vi "Convert CAN Log Files.vi"() -> ()   [LabVIEW 2010, in "CAN Log Transfer and Convert.lvlib"]
uses:
  CAN Log Transfer and Convert.lvlib
  NICAN Warning.ctl
  Stop FGV Commands.ctl
  Global.vi
panel:
  out "CAN Warning":T1=TRUE
  in  "Text format":enum32{"NI-CAN", "NI-XNET"}(radio)
  in  "Destination directory":path
  in  "Recursive?":bool=TRUE
  in  "Directory of NCL files":path
  out "Progress":u8(slide) scale=0.0..100.0
  in  "Abort":bool
  in  "Start":bool
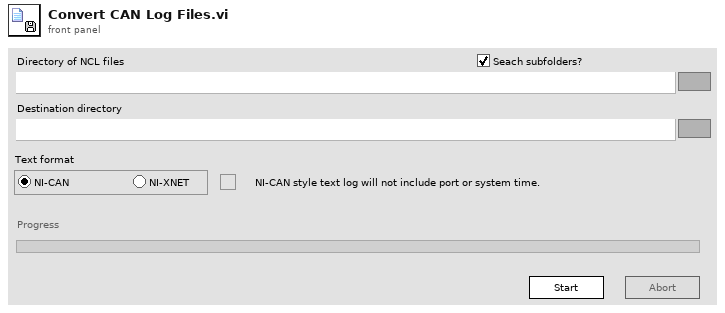
[diagram p1: front panel]
types:
  T1 = typedef "CAN Log Transfer and Convert.lvlib/NICAN Warning.ctl" = bool
  T2 = typedef "CAN Log Transfer and Convert.lvlib/Stop FGV Commands.ctl" = enum16{"Write", "Read", "Reset"}
  T3 = enum8{"Enabled", "Disabled", "Disabled and Grayed Out"}
  T4 = enum32{"invalid app kind", "Development System", "Run Time System", "Student Edition", "Embedded LabVIEW", "Evaluation", "Custom"}
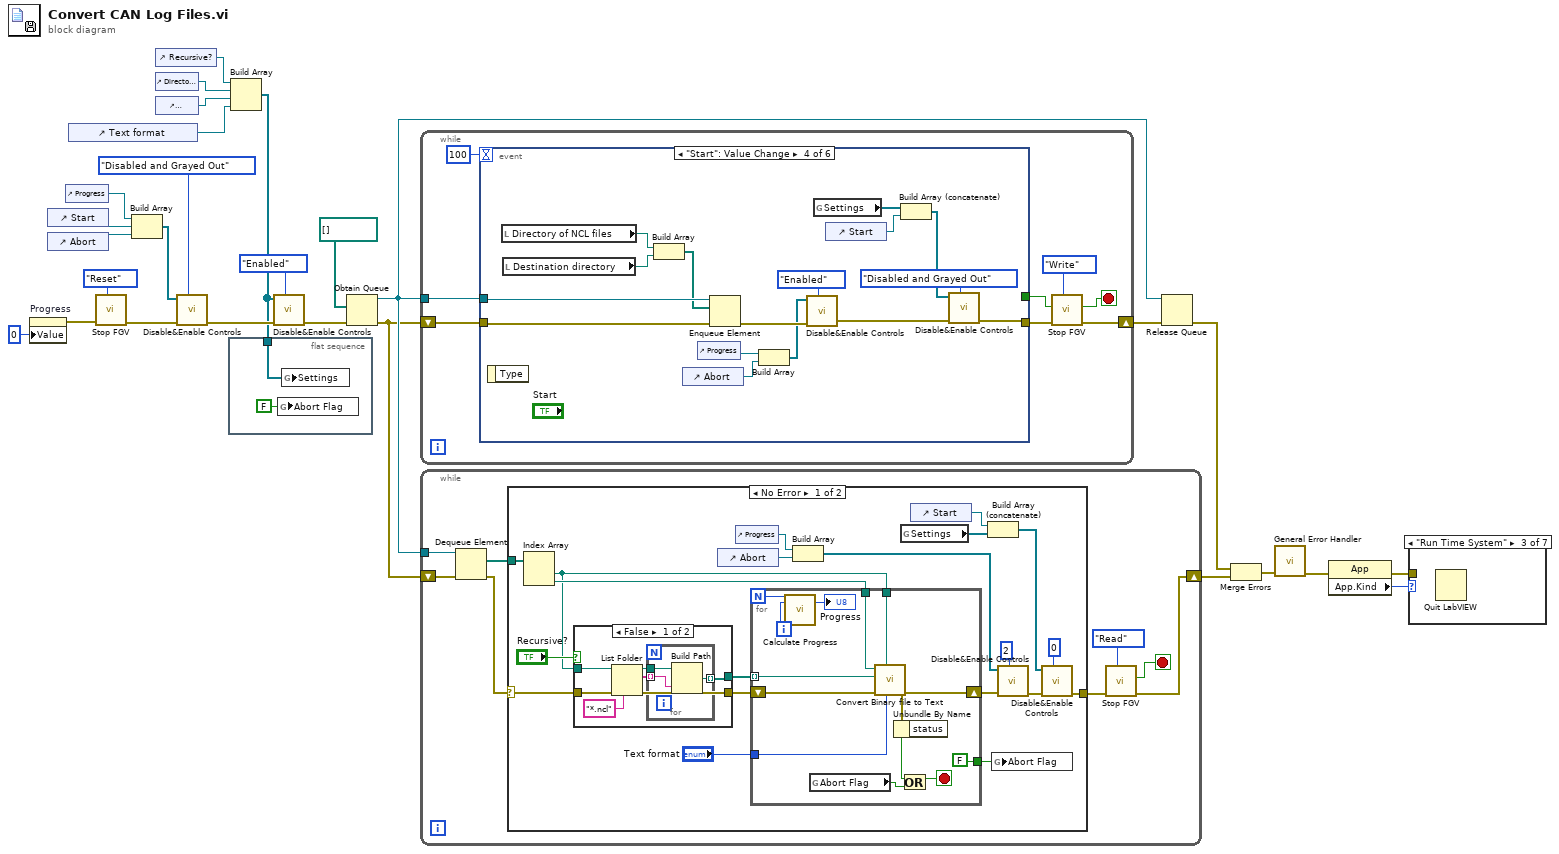
[diagram p0: block diagram]
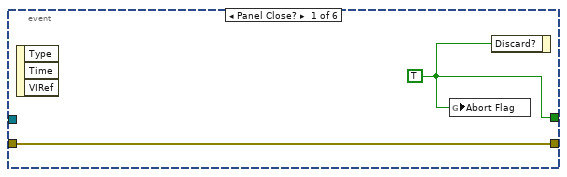
[diagram p8: hidden frame]
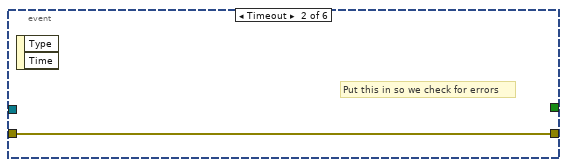
[diagram p9: hidden frame]
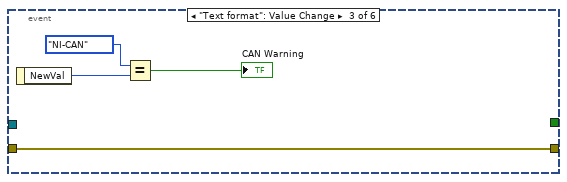
[diagram p10: hidden frame]
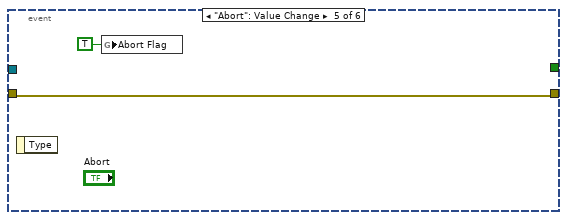
[diagram p11: hidden frame]
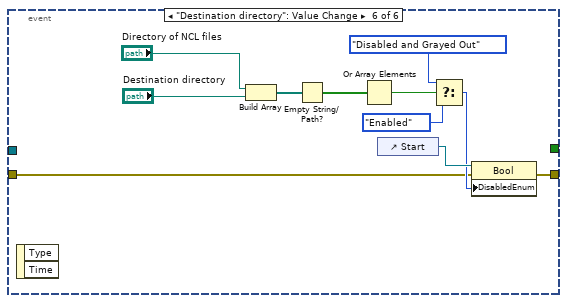
[diagram p12: hidden frame]
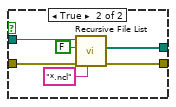
[diagram p13: hidden frame]
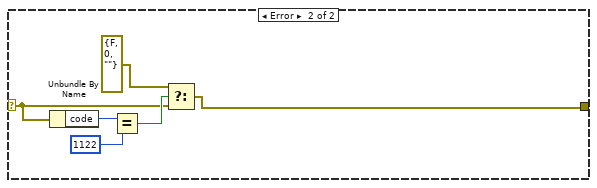
[diagram p14: hidden frame]
diagram:
  n1 = property on="Progress" class="Slide (strict)"("Value"=u8 0 ("Progress")) -> (error out=w8:errorcluster)  [unwired: 2 in, 1 out]
  n2 = control-ref of="Start"() -> (w21:refnum<vi>)
  n3 = control-ref of="Abort"() -> (w20:refnum<vi>)
  n4 = control-ref of="Progress"() -> (w22:refnum<vi>)
  n5 = control-ref of="Text format"() -> (w1:refnum<vi>)
  n6 = call "Stop FGV.vi"("Command"=Stop_FGV_Commands."Reset", "error in (no error)"=w8) -> ("error out"=w4:errorcluster)  [unwired: 7 in, 2 out]
  n7 = Build Array(w22, w21, w20) -> (w19:refnum<vi>[])
  n8 = control-ref of="Recursive?"() -> (w25:refnum<vi>)
  n9 = control-ref of="Directory of NCL files"() -> (w26:refnum<vi>)
  n10 = control-ref of="Destination directory"() -> (w27:refnum<vi>)
  n11 = call "Disable&Enable Controls.vi"("State"=T3."Disabled and Grayed Out", "error in (no error)"=w4, "Controls"=w19) -> ("error out"=w23:errorcluster)  [unwired: 8 in]
  n12 = flat-sequence {
    tunnel: w3 -> [w28]
    frame #0 {
      n13 = global write "Global.vi" "Abort Flag"(FALSE) -> ()
      n14 = global write "Global.vi" "Settings"(w28) -> ()
    }
  }
  n15 = Build Array(w25, w26, w27, w1) -> (w3:refnum<vi>[])
  n16 = call "Disable&Enable Controls.vi"("State"=T3."Enabled" ("Disabled"), "error in (no error)"=w23, "Controls"=w3) -> ("error out"=w17:errorcluster)  [unwired: 8 in]
  n17 = Obtain Queue(element data type=path[] [], error in (no error)=w17) -> (queue out=w13:refnum<queue>, error out=w12:errorcluster)  [unwired: 3 in, 1 out]
  n18 = while {
    shift-right: [w34] -> w15
    shift-left: w12 -> [w37]
    tunnel: w13 -> [w36]
    stop <- w33 stop-if-true
    n19 = event shown="[3] \"Start\": Value Change" {
      selector: _ -> [_ _ _ _ _ _]
      dyn-events: _ -> [_ _ _ _ _ _]
      timeout: 100 -> [_ _ _ _ _ _]
      tunnel: [w38 _ _ _ _ _] -> w31
      tunnel: w37 -> [w39 w40 w41 w60 w61 w63]
      tunnel: [w39 w40 w41 w52 w61 w67] -> w35
      tunnel: w36 -> [_ _ _ w59 _ _]
      event Panel Close? {
        w38 = TRUE
        n20 = event-data() -> ()  [unwired: 1 in, 3 out]
        n21 = global write "Global.vi" "Abort Flag"(w38) -> ()
        n22 = event-data("Discard?"=w38) -> ()  [unwired: 1 in, 1 out]
      }
      event Timeout {
        # "Put this in so we check for errors"
        n23 = event-data() -> ()  [unwired: 1 in, 2 out]
      }
      event "Text format": Value Change {
        n24 = event-data() -> ("NewVal"=w44:enum32{"NI-CAN", "NI-XNET"})  [unwired: 1 in]
        n25 = Equal?(x=enum32{"NI-CAN", "NI-XNET"}."NI-CAN", y=w44) -> (x = y?=→"CAN Warning":bool)
      }
      event "Start": Value Change {
        n26 = event-data() -> ()  [unwired: 1 in, 1 out]
        n27 = local read "Directory of NCL files"() -> (w58:path)
        n28 = local read "Destination directory"() -> (w45:path)
        n29 = Build Array(w58, w45) -> (w57:path[])
        n30 = control-ref of="Abort"() -> (w51:refnum<vi>)
        n31 = control-ref of="Progress"() -> (w50:refnum<vi>)
        n32 = Enqueue Element(queue=w59, element=w57, error in (no error)=w60) -> (error out=w56:errorcluster)  [unwired: 1 in, 2 out]
        n33 = Build Array(w50, w51) -> (w49:refnum<vi>[])
        n34 = call "Disable&Enable Controls.vi"("State"=T3."Enabled", "error in (no error)"=w56, "Controls"=w49) -> ("error out"=w54:errorcluster)  [unwired: 8 in]
        n35 = global read "Global.vi" "Settings"() -> (w46:refnum<vi>[])
        n36 = control-ref of="Start"() -> (w48:refnum<vi>)
        n37 = Build Array (concatenate)(w46, w48) -> (w47:refnum<vi>[])
        n38 = call "Disable&Enable Controls.vi"("State"=T3."Disabled and Grayed Out", "error in (no error)"=w54, "Controls"=w47) -> ("error out"=w52:errorcluster)  [unwired: 8 in]
      }
      event "Abort": Value Change {
        n39 = event-data() -> ()  [unwired: 1 in, 1 out]
        n40 = global write "Global.vi" "Abort Flag"(TRUE ("Abort Flag")) -> ()
      }
      event "Destination directory": Value Change {
        n41 = event-data() -> ()  [unwired: 1 in, 2 out]
        n42 = Build Array("Directory of NCL files", "Destination directory") -> (w71:path[])
        n43 = Empty String/Path?(string/path=w71) -> (empty?=w64:bool[])
        n44 = Or Array Elements(Boolean array=w64) -> (logical OR=w70:bool)
        n45 = control-ref of="Start"() -> (w66:refnum<vi>)
        n46 = Select(t=T3."Disabled and Grayed Out" ("State"), s=w70, f=T3."Enabled") -> (s? t:f=w65:T3)
        n47 = property class="Bool"(reference=w66, error in=w63, "DisabledEnum"=w65) -> (error out=w67:errorcluster)  [unwired: 1 out]
      }
    }
    n48 = call "Stop FGV.vi"("Command"=Stop_FGV_Commands."Write", "error in (no error)"=w35, "Stop?"=w31) -> ("error out"=w34:errorcluster, "Latched Stop"=w33:bool)  [unwired: 6 in, 1 out]
  }
  n49 = while {
    shift-right: [w78] -> w10
    shift-left: w12 -> [w81]
    tunnel: w13 -> [w80]
    stop <- w77 stop-if-true
    n50 = Dequeue Element(queue=w80, error in (no error)=w81) -> (element=w75:path[], error out=w79:errorcluster)  [unwired: 1 in, 2 out]
    n51 = case shown="No Error" w79 {
      selector: w79 -> [w82 w133]
      tunnel: [w96 w132] -> w74
      tunnel: w75 -> [w92 _]
      frame No Error {
        n52 = Index Array(array=w92) -> (element #1=w84:path, element #2=w86:path)  [unwired: 2 in]
        n53 = case shown="False" "Recursive?" {
          tunnel: w84 -> [w120 w130]
          tunnel: w82 -> [w121 w127]
          tunnel: [w117 w126] -> w90
          tunnel: [w115 w125] -> w89
          frame False {
            n54 = List Folder(path=w120, pattern="*.ncl", error in=w121) -> (path out=w119:path, filenames=w118:string[], error out=w117:errorcluster)  [unwired: 1 in, 1 out]
            n55 = for {
              tunnel: w119 -> [w124]
              tunnel: w118 -> [w123] mode=indexing
              tunnel: [w122] -> w115 mode=indexing
              n56 = Build Path(base path=w124, name or relative path=w123) -> (appended path=w122:path)
            }
          }
          frame True {
            n57 = call <vilib>:"Recursive File List.vi"("pattern"="*.ncl", "error in (no error)"=w127, "Treat LLBs as Folders?"=FALSE, "Folder Path"=w130) -> ("error out"=w126:errorcluster, "All Files in Dir"=w125:path[])  [unwired: 3 in, 3 out]
          }
        }
        n58 = control-ref of="Abort"() -> (w99:refnum<vi>)
        n59 = control-ref of="Progress"() -> (w100:refnum<vi>)
        n60 = for {
          N -> [w112]
          tunnel: w89 -> [w105] mode=indexing
          shift-right: [w102] -> w88
          shift-left: w90 -> [w109]
          tunnel: [FALSE] -> w87
          tunnel: w86 -> [w108]
          tunnel: w84 -> [w107]
          tunnel: "Text format" -> [w106]
          i -> [w113]
          stop <- w104 stop-if-true
          n61 = call "Calculate Progress.vi"("Total Iterations"=w112, "Current Iteration"=w113) -> ("Progress"=→"Progress":u8)  [unwired: 17 in]
          n62 = global read "Global.vi" "Abort Flag"() -> (w110:bool)
          n63 = call "Convert Binary file to Text.vi"("Text format"=w106, "Originating directory"=w107, "error in (no error)"=w109, "NCL File Path"=w105, "Destination directory"=w108) -> ("error out"=w102:errorcluster)  [unwired: 6 in]
          n64 = Unbundle By Name(w102) -> ("status"=w103:bool)
          n65 = Or(x=w103, y=w110) -> (x .or. y?=w104:bool)
        }
        n66 = Build Array(w100, w99) -> (w98:refnum<vi>[])
        n67 = global read "Global.vi" "Settings"() -> (w85:refnum<vi>[])
        n68 = control-ref of="Start"() -> (w94:refnum<vi>)
        n69 = Build Array (concatenate)(w94, w85) -> (w93:refnum<vi>[])
        n70 = global write "Global.vi" "Abort Flag"(w87) -> ()
        n71 = call "Disable&Enable Controls.vi"("State"=2, "error in (no error)"=w88, "Controls"=w98) -> ("error out"=w97:errorcluster)  [unwired: 8 in]
        n72 = call "Disable&Enable Controls.vi"("State"=0, "error in (no error)"=w97, "Controls"=w93) -> ("error out"=w96:errorcluster)  [unwired: 8 in]
      }
      frame Error {
        n73 = Unbundle By Name(w133) -> ("code"=w136:i32)
        n74 = Equal?(x=w136, y=1122) -> (x = y?=w134:bool)
        n75 = Select(t=errorcluster {"status"=FALSE, "code"=0, "source"=""}, s=w134, f=w133) -> (s? t:f=w132:errorcluster)
      }
    }
    n76 = call "Stop FGV.vi"("Command"=Stop_FGV_Commands."Read", "error in (no error)"=w74) -> ("error out"=w78:errorcluster, "Latched Stop"=w77:bool)  [unwired: 7 in, 1 out]
  }
  n77 = Release Queue(queue=w13, error in (no error)=w15) -> (error out=w14:errorcluster)  [unwired: 1 in, 2 out]
  n78 = Merge Errors(w14, w10) -> (w9:errorcluster)
  n79 = call <vilib>:"General Error Handler.vi"("error in (no error)"=w9) -> ("error out"=w6:errorcluster)  [unwired: 10 in, 4 out]
  n80 = property class="App"(error in=w6) -> (error out=w2:errorcluster, "App.Kind"=w5:T4)  [unwired: 1 in, 1 out]
  n81 = case shown="\"Run Time System\"" w5 {
    tunnel: w2 -> [_ _ _ _ _ _ _]
    frame "invalid app kind", Default {
    }
    frame "Development System" {
    }
    frame "Run Time System" {
      n82 = Quit LabVIEW() -> ()  [unwired: 1 in]
    }
    frame "Student Edition" {
    }
    frame "Embedded LabVIEW" {
    }
    frame "Evaluation" {
    }
    frame "Custom" {
    }
  }
